vi "4.3.vi"() -> ()   [LabVIEW 2017]
panel:
  out "平方根":dbl
  in  "输入值":dbl
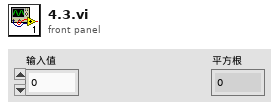
[diagram p1: front panel]
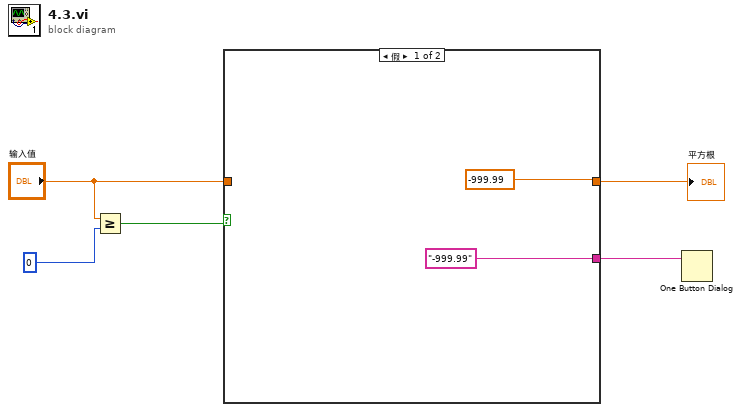
[diagram p0: block diagram]
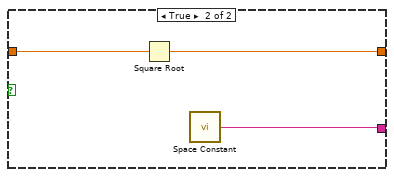
[diagram p2: hidden frame]
diagram:
  n1 = Greater Or Equal?(x="输入值", y=0) -> (x >= y?=w4:bool)
  n2 = case shown="假" w4 {
    tunnel: ["-999.99" w8] -> w3
    tunnel: "输入值" -> [_ w10]
    tunnel: [-999.99 w9] -> w1
    frame False {
    }
    frame True {
      n3 = Square Root(x=w10) -> (sqrt(x)=w9:dbl)
      n4 = call <vilib>:"Space Constant.vi"() -> ("String"=w8:string)
    }
  }
  "平方根" <- w1
  n5 = One Button Dialog(message=w3) -> ()  [unwired: 1 in, 1 out]
